vi "HMF2500 Initialize.vi"(7 "Serial Configuration":T1={"Baud Rate"=9600, "Parity"=0, "Data Bits"=8, "Flow Control"=4} {"Flow Control" items=["None", "XON/XOFF", "RTS/CTS", "XON/XOFF & RTS/CTS", "DTR/DSR", "XON/XOFF & DTR/DSR"]; "Data Bits" items=["7"=7, "8"=8]; "Parity" items=["None", "Odd", "Even", "Mark", "Space"]; "Baud Rate" items=["300"=300, "600"=600, "1200"=1200, "2400"=2400, "4800"=4800, "9600"=9600, "19200"=19200]}, 8 "error in (no error)":errorcluster, 9 "Reset (True)":bool=TRUE, 10 "ID Query (True)":bool=TRUE, 11 "VISA resource name":refnum<visa-resource-name>) -> (0 "error out":errorcluster, 2 "idn string":string, 3 "VISA resource name out":refnum<visa-resource-name>)   [LabVIEW 2020, in "AWG.lvlib"]
doc: "Establishes communication with the instrument and optionally performs an instrument identification query and/or an instrument reset. It also places the instrument in a default state needed for other instrument driver operations. Therefore, call this VI before calling other instrument driver VIs for this instrument. Generally, you need to call the <B>Initialize VI</B> only once at the beginning of an application."
uses:
  AWG.lvlib
panel:
  # "(c) 2005- 2013 National Instruments.  ALL RIGHTS RESERVED."
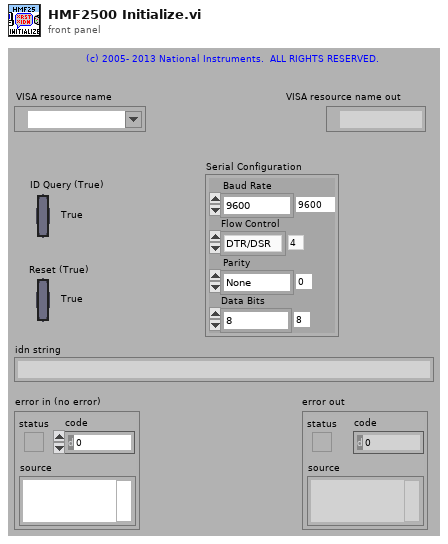
[diagram p1: front panel]
types:
  T1 = cluster{"Baud Rate":u32, "Parity":u16, "Data Bits":u16, "Flow Control":u16}
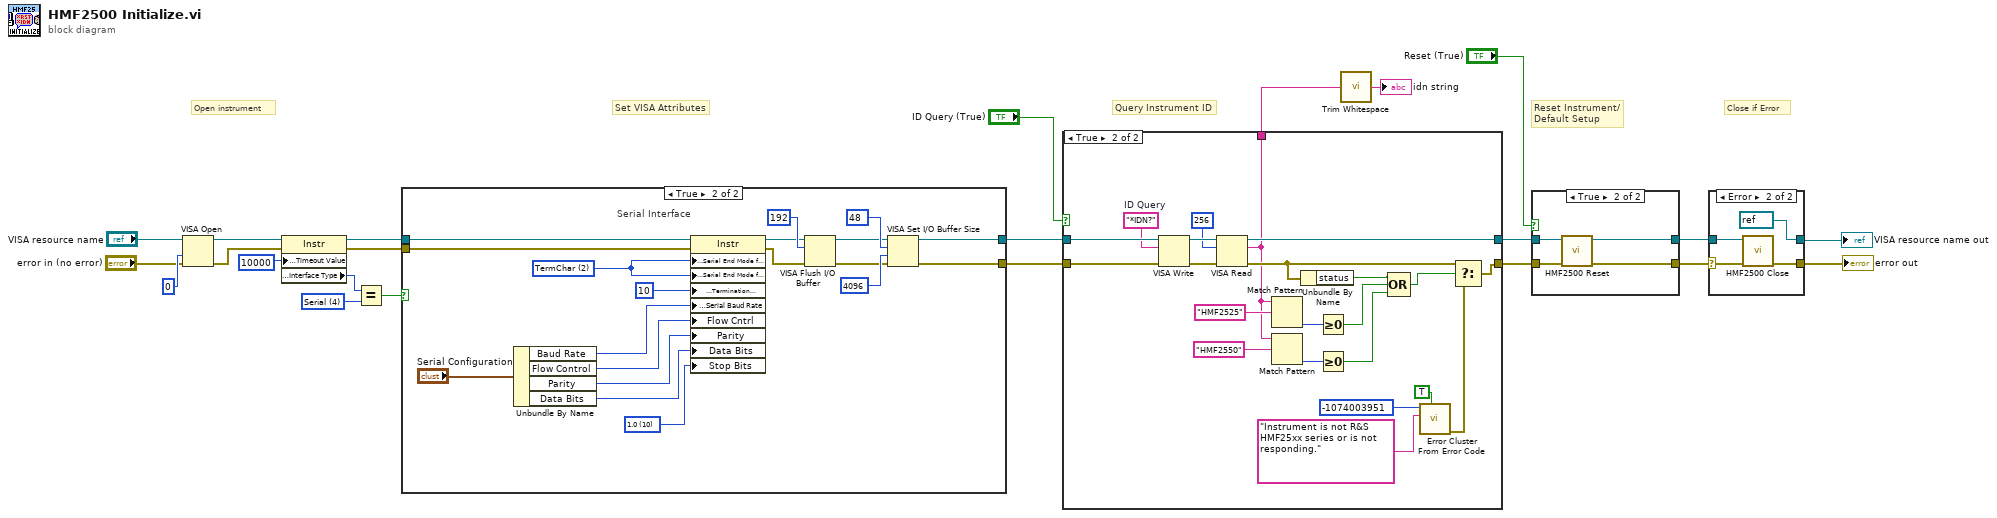
[diagram p0: block diagram]
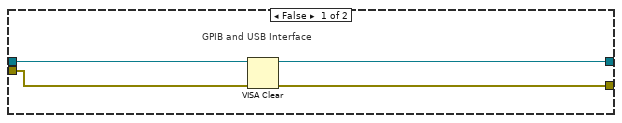
[diagram p2: hidden frame]
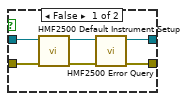
[diagram p4: hidden frame]
diagram:
  w16 = u16 4 items=["GPIB"=1, "VXI"=2, "GPIB-VXI"=3, "Serial"=4, "PXI"=5, "TCPIP"=6, "USB"=7] ("Interface Information:Interface Type")
  # "Set VISA Attributes"
  # "Close if Error"
  # "Query Instrument ID"
  # "Reset Instrument/\nDefault Setup"
  # "Open instrument"
  n1 = VISA Open(access mode=u32 0, error in (no error)="error in (no error)", VISA resource name="VISA resource name") -> (VISA resource name=w13:refnum<visa-resource-name>, error out=w12:errorcluster)  [unwired: 2 in]
  n2 = property class="Instr"(reference=w13, error in=w12, "General Settings:Timeout Value"=u32 10000) -> (reference out=w19:refnum<visa-resource-name>, error out=w18:errorcluster, "Interface Information:Interface Type"=w23:u16)
  n3 = Equal?(x=w23, y=w16) -> (x = y?=w17:bool)
  n4 = case shown="True" w17 {
    tunnel: [w25 w30] -> w21
    tunnel: [w24 w29] -> w20
    tunnel: w19 -> [w27 w45]
    tunnel: w18 -> [w26 w46]
    frame False {
      # "GPIB and USB Interface"
      n5 = VISA Clear(VISA resource name=w27, error in (no error)=w26) -> (VISA resource name out=w25:refnum<visa-resource-name>, error out=w24:errorcluster)
    }
    frame True {
      w32 = u16 10 items=["1.0"=10, "1.5"=15, "2.0"=20] ("Serial Settings:Stop Bits")
      w44 = u16 2 items=["None", "LastBit", "TermChar"] ("Serial Settings:Serial End Mode for Reads")
      # "Serial Interface"
      n6 = Unbundle By Name("Serial Configuration") -> ("Baud Rate"=w42:u32, "Flow Control"=w31:u16, "Parity"=w41:u16, "Data Bits"=w40:u16)
      n7 = property class="Instr"(reference=w45, error in=w46, "Serial Settings:Serial End Mode for Reads"=w44, "Serial Settings:Serial End Mode for Writes"=w44, "Message Based Settings:Termination Character"=u8 10, "Serial Settings:Serial Baud Rate"=w42, "Flow Cntrl"=w31, "Parity"=w41, "Data Bits"=w40, "Stop Bits"=w32) -> (reference out=w38:refnum<visa-resource-name>, error out=w37:errorcluster)
      n8 = VISA Flush I/O Buffer(VISA resource name=w38, mask (16)=u16 192, error in (no error)=w37) -> (VISA resource name out=w33:refnum<visa-resource-name>, error out=w34:errorcluster)
      n9 = VISA Set I/O Buffer Size(VISA resource name=w33, mask (16)=u16 48, size (4096)=u32 4096 ("size (0)"), error in (no error)=w34) -> (VISA resource name out=w30:refnum<visa-resource-name>, error out=w29:errorcluster)
    }
  }
  n10 = case shown="True" "ID Query (True)" {
    tunnel: [w47 w70] -> w2
    tunnel: [w48 w67] -> w1
    tunnel: w21 -> [w48 w68]
    tunnel: w20 -> [w47 w69]
    tunnel: [_ w49] -> w4
    frame False {
    }
    frame True {
      w62 = "*IDN?"  # ID Query
      n11 = VISA Write(VISA resource name=w68, write buffer=w62, error in (no error)=w69) -> (VISA resource name out=w66:refnum<visa-resource-name>, error out=w65:errorcluster)  [unwired: 1 out]
      n12 = VISA Read(VISA resource name=w66, byte count=u32 256, error in (no error)=w65) -> (VISA resource name out=w67:refnum<visa-resource-name>, read buffer=w49:string, error out=w56:errorcluster)  [unwired: 1 out]
      n13 = Match Pattern(string=w49, regular expression="HMF2525") -> (offset past match=w64:i32)  [unwired: 1 in, 3 out]
      n14 = Match Pattern(string=w49, regular expression="HMF2550") -> (offset past match=w51:i32)  [unwired: 1 in, 3 out]
      n15 = Unbundle By Name(w56) -> ("status"=w55:bool)
      n16 = Greater Or Equal To 0?(x=w64) -> (x >= 0?=w54:bool)
      n17 = Greater Or Equal To 0?(x=w51) -> (x >= 0?=w53:bool)
      n18 = Compound Arithmetic op=OR(w55, w54, w53) -> (w52:bool)
      n19 = call <vilib>:"Error Cluster From Error Code.vi"("show call chain? (False)"=TRUE, "error message (\"\")"="Instrument is not R&S HMF25xx series or is not responding." ("Source (VI Name)"), "error code (0)"=-1074003951 ("Code")) -> ("error out"=w61:errorcluster)  [unwired: 6 in]
      n20 = Select(t=w56, s=w52, f=w61) -> (s? t:f=w70:errorcluster)
    }
  }
  n21 = call <vilib>:"Trim Whitespace.vi"("string"=w4) -> ("trimmed string"=→"idn string":string)  [unwired: 1 in]
  n22 = case shown="True" "Reset (True)" {
    tunnel: [w73 w80] -> w14
    tunnel: [w74 w79] -> w15
    tunnel: w2 -> [w72 w77]
    tunnel: w1 -> [w71 w78]
    frame False {
      n23 = call "HMF2500 Default Instrument Setup.vi"("error in (no error)"=w72, "VISA resource name"=w71) -> ("error out"=w75:errorcluster, "VISA resource name out"=w76:refnum<visa-resource-name>)  [unwired: 8 in]
      n24 = call "HMF2500 Error Query.vi"("error in (no error)"=w75, "VISA resource name"=w76) -> ("error out"=w73:errorcluster, "VISA resource name out"=w74:refnum<visa-resource-name>)  [unwired: 6 in, 2 out]
    }
    frame True {
      n25 = call "HMF2500 Reset.vi"("error in (no error)"=w77, "VISA resource name"=w78) -> ("error out"=w80:errorcluster, "VISA resource name out"=w79:refnum<visa-resource-name>)  [unwired: 8 in]
    }
  }
  n26 = case shown="Error" w14 {
    selector: w14 -> [w81 w84]
    tunnel: w15 -> [w82 w85]
    tunnel: [w82 refnum<visa-resource-name> refnum ("VISA resource name out")] -> w9
    tunnel: [w81 w86] -> w8
    frame No Error {
    }
    frame Error {
      n27 = call "HMF2500 Close.vi"("error in (no error)"=w84, "VISA resource name"=w85) -> ("error out"=w86:errorcluster)  [unwired: 9 in]
    }
  }
  "VISA resource name out" <- w9
  "error out" <- w8
